vi "UIRef.vi"(8 "error in":errorcluster, 11 "cRIO in":refnum<class "PLTarget cRIO.lvclass">) -> (0 "error out":errorcluster, 2 "VI refnum":refnum<vi>, 3 "cRIO out":refnum<class "PLTarget cRIO.lvclass">)   [LabVIEW 2013, in "PLTarget cRIO.lvclass"]
uses:
  PLTarget cRIO.lvclass
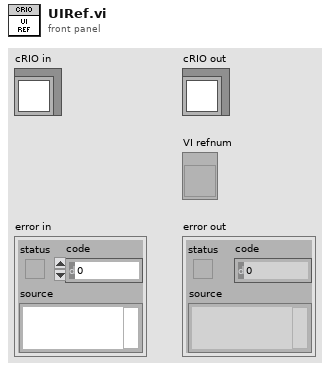
[diagram p1: front panel]
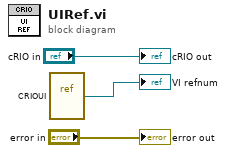
[diagram p0: block diagram]
diagram:
  n1 = vi-ref "CRIOUI.vi"() -> (→"VI refnum":refnum<vi>)
  "error out" <- "error in"
  "cRIO out" <- "cRIO in"
